vi "State_Machine.vi"(8 "error in (no error)":errorcluster caption="entrée d'erreur (pas d'erreur)", 11 "Nodon_Get_BP_Status IN":refnum<class "Nodon_Get_Switch_Status.lvclass">) -> (0 "error out":errorcluster caption="sortie d'erreur", 2 "Json_String":string, 3 "Nodon_Get_BP_Status OUT":refnum<class "Nodon_Get_Switch_Status.lvclass">)   [LabVIEW 2020, in "Library Test.lvlib" / "Nodon_Get_Switch_Status.lvclass"]
uses:
  Nodon_Get_Switch_Status.lvclass
  C:/Users/ngarcin/OneDrive - Altyor/Standard TB/Class/Test/Test (Default)/Test (Default).lvclass
  C:/Users/ngarcin/OneDrive - Altyor/Standard TB/Class/Test/Nodon_Send_Command_UART/Nodon_Send_Command_UART.lvclass
  JSON API/JSON Value/Set from JSON string.vi
  JSON API/JSON Value/JSON Value.lvclass
  Nodon_Send_Command_UART/Nodon_Send_Command_UART.lvclass
  Nodon_Get_Switch_Status.lvclass/Nodon_Get_Switch_Status.ctl
  JSON API/Variant JSON/Variant JSON.lvlib
  JSON API/Get Polymorphic/JSON GetSet.lvlib
  Commun VI/Library Commun.lvlib
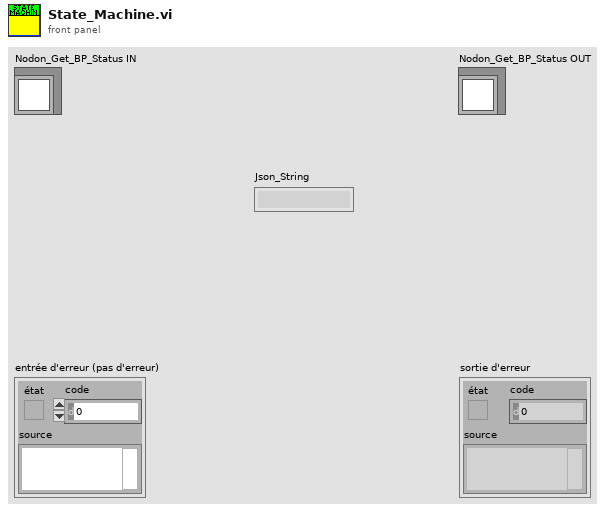
[diagram p1: front panel]
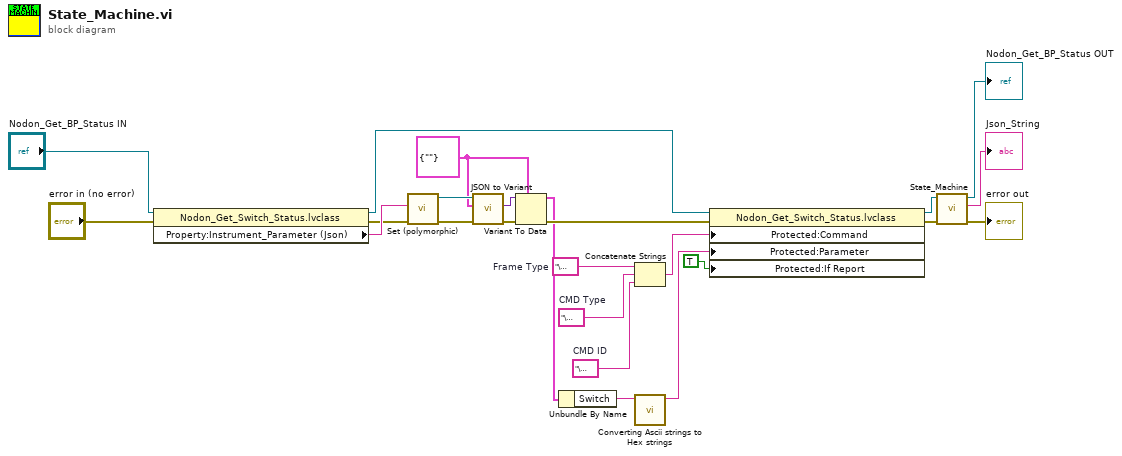
[diagram p0: block diagram]
diagram:
  w8 = cluster{"Switch":string} {"Switch"=""}
  w19 = "\u0000"  # Frame Type
  w18 = "\u0003"  # CMD ID
  w17 = "\u0001"  # CMD Type
  n1 = property class="Nodon_Get_Switch_Status.lvclass"(reference="Nodon_Get_BP_Status IN", error in="error in (no error)") -> (reference out=w6:refnum<class "Nodon_Get_Switch_Status.lvclass">, error out=w9:errorcluster, "Property:Instrument_Parameter (Json)"=w10:string)
  n2 = call-poly "Set (polymorphic).vi"("error in (no error)"=w9, "JSON stream"=w10) -> ("error out"=w12:errorcluster, "JSON Value out"=w14:refnum<class "JSON Value.lvclass">)  [unwired: 7 in, 1 out]
  n3 = call "JSON to Variant.vi"("error in (no error)"=w12, "Variant (Data Type)"=w8, "JSON Value"=w14) -> ("error out"=w13:errorcluster, "Variant out"=w11:variant)  [unwired: 7 in]
  n4 = Variant To Data(error in=w13, type=w8, Variant=w11) -> (data=w3:cluster{"Switch":string}, error out=w4:errorcluster)
  n5 = Unbundle By Name(w3) -> ("Switch"=w2:string)
  n6 = Concatenate Strings(w19, w17, w18) -> (w16:string)
  n7 = call "Converting Ascii strings to Hex strings.vi"("result string"=w2) -> ("Chaîne"=w1:string)  [unwired: 10 in]
  n8 = property class="Nodon_Get_Switch_Status.lvclass"(reference=w6, error in=w4, "Protected:Command"=w16, "Protected:Parameter"=w1, "Protected:If Report"=TRUE ("If Report")) -> (reference out=w21:refnum<class "Nodon_Get_Switch_Status.lvclass">, error out=w20:errorcluster)
  n9 = call-parent "State_Machine.vi"("error in (no error)"=w20, "Send_Frame en entrée"=w21) -> ("error out"=→"error out":errorcluster, "Json_String"=→"Json_String":string, "Send_Frame en sortie"=→"Nodon_Get_BP_Status OUT":refnum<class "Nodon_Get_Switch_Status.lvclass">)  [unwired: 7 in]
